vi "Pop-up wait prompt.vi"(8 "error in (no error)":errorcluster, 9 "Prompt Text":string, 10 "Is Dialog?":enum16{"Normal", "Dialog Box"}(ring), 11 "Control":enum16{"Open", "Close", "Status", "No Change"}(ring)) -> (0 "error out":errorcluster)   [LabVIEW 2013, in "GUI.lvlib"]
doc: "If there is no error in, this vi will either open or close the calling panel which displays a prompt to wait. The input control determines whether the panel is opened or closed. Typically called before intensive processing with control=open and after with control = close.\n\nClose action ignores error in."
uses:
  GUI.lvlib
  <vilib>/Utility/miscctls.llb/LVPointTypeDef.ctl
  Timing/Timing Lib.lvlib
panel:
  out "Prompt":string
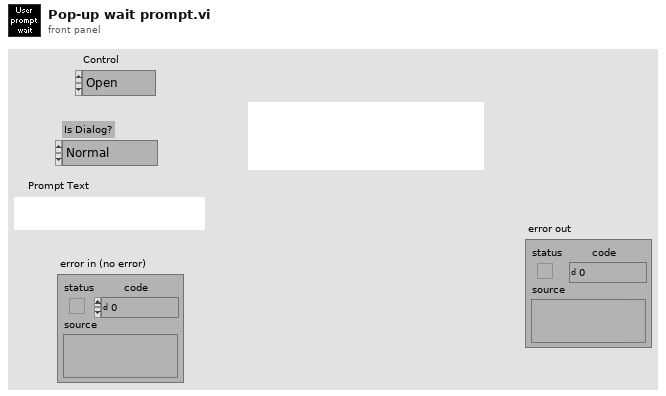
[diagram p1: front panel]
types:
  T1 = typedef "LVPointTypeDef.ctl" = cluster{"Horizontal":i16, "Vertical":i16}
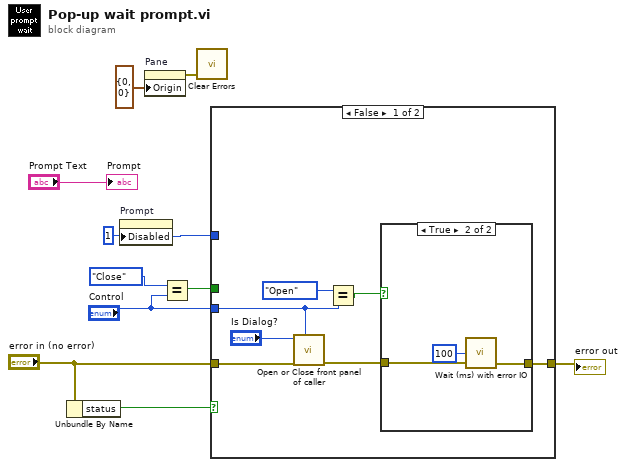
[diagram p0: block diagram]
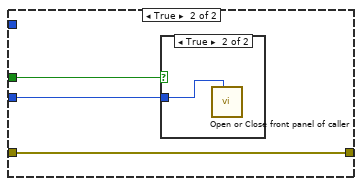
[diagram p3: hidden frame]
diagram:
  w4 = u8 1 ("Write Attribute")
  n1 = Unbundle By Name("error in (no error)") -> ("status"=w8:bool)
  n2 = property on="Prompt" class="Str"("Disabled"=w4) -> ()  [unwired: 2 in, 2 out]
  n3 = property on="Pane" class="Pane"("Origin"=T1 {"Horizontal"=0, "Vertical"=0}) -> (error out=w1:errorcluster)  [unwired: 2 in, 1 out]
  n4 = Equal?(x=enum16{"Open", "Close", "Status", "No Change"}."Close", y="Control") -> (x = y?=w6:bool)
  n5 = call <vilib>:"Clear Errors.vi"("error in (no error)"=w1) -> ()  [unwired: 6 in, 1 out]
  n6 = case shown="False" w8 {
    tunnel: [w12 w24] -> w10
    tunnel: "error in (no error)" -> [w17 w24]
    tunnel: w6 -> [_ w23]
    tunnel: "Control" -> [w16 w22]
    tunnel: w4 -> [_ _]
    frame False {
      n7 = call "Open or Close front panel of caller.vi"("Control"=w16, "error in (no error)"=w17, "Is Dialog?"="Is Dialog?") -> ("error out"=w13:errorcluster)  [unwired: 3 in, 3 out]
      n8 = Equal?(x=enum16{"Open", "Close", "Status", "No Change"}."Open", y=w16) -> (x = y?=w14:bool)
      n9 = case shown="True" w14 {
        tunnel: w13 -> [w18 w21]
        tunnel: [w18 w20] -> w12
        frame False {
        }
        frame True {
          n10 = call "Wait (ms) with error IO.vi"("error in (no error)"=w21, "milliseconds to wait"=u32 100) -> ("error out"=w20:errorcluster)  [unwired: 3 in]
        }
      }
    }
    frame True {
      n11 = case shown="True" w23 {
        tunnel: w22 -> [_ w25]
        frame False {
        }
        frame True {
          n12 = call "Open or Close front panel of caller.vi"("Control"=w25) -> ()  [unwired: 5 in, 4 out]
        }
      }
    }
  }
  "error out" <- w10
  "Prompt" <- "Prompt Text"
